vi "DateIntToDateMMDDYYYY.vi"() -> ()   [LabVIEW 2009]
panel:
  out "Year":u32
  out "Month":u32
  out "Day":u32
  in  "Date Int":u16
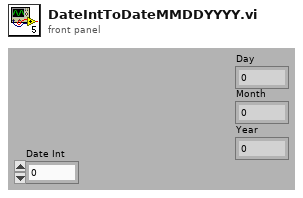
[diagram p1: front panel]
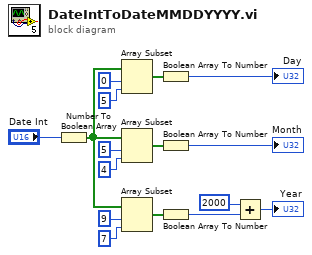
[diagram p0: block diagram]
diagram:
  n1 = Number To Boolean Array(number="Date Int") -> (Boolean array=w3:bool[])
  n2 = Array Subset(array=w3, index=0, length=5) -> (w13:bool[])
  n3 = Array Subset(array=w3, index=5, length=4) -> (w9:bool[])
  n4 = Array Subset(array=w3, index=9, length=7) -> (w5:bool[])
  n5 = Boolean Array To Number(Boolean array=w13) -> (number=→"Day":u32)
  n6 = Boolean Array To Number(Boolean array=w9) -> (number=→"Month":u32)
  n7 = Boolean Array To Number(Boolean array=w5) -> (number=w4:u32)
  n8 = Add(x=u32 2000, y=w4) -> (x+y=→"Year":u32)
